vi "kSARegisterForData.vi"(0 "kSAComm ref in":refnum<k24>, 1 "Data Definitions":T1(array[cluster])) -> (2 "kSAComm ref out":refnum<k24>, 3 "Success":bool, 4 "Error":string)   [LabVIEW 2019]
doc: "Set up the kSA Data Store with the desired data items to retrieve when syncing data with the kSA Application."
uses:
  C:/Users/tim/Documents/kSAComm LabView Sample/kSACommInterface.dll
  kSACommInterface.dll
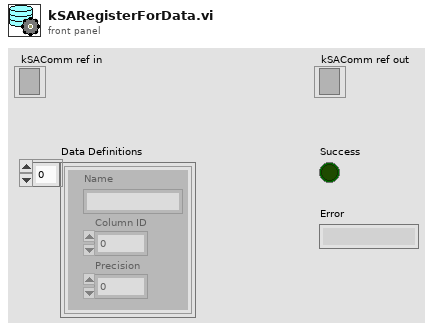
[diagram p1: front panel]
types:
  T1 = cluster{"Name":string, "Column ID":u32, "Precision":i32}[]
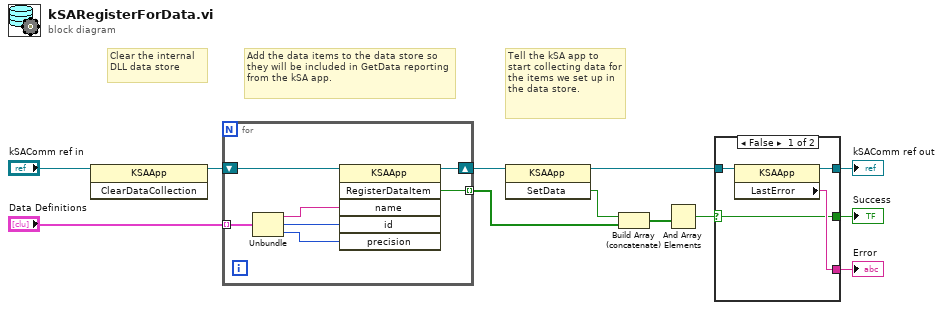
[diagram p0: block diagram]
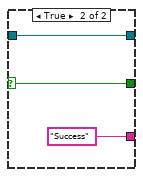
[diagram p2: hidden frame]
diagram:
  # "Add the data items to the data store so they will be included in GetData reporting from the kSA app."
  # "Clear the internal DLL data store"
  # "Tell the kSA app to start collecting data for the items we set up in the data store."
  n1 = invoke class="KSAApp" method="ClearDataCollection"(reference="kSAComm ref in") -> (reference out=w10:refnum<k24>)  [unwired: 2 in, 2 out]
  n2 = for {
    shift-right: [w14] -> w9
    shift-left: w10 -> [w15]
    tunnel: "Data Definitions" -> [w19] mode=indexing
    tunnel: [w13] -> w7 mode=indexing
    n3 = Unbundle(w19) -> ("Name"=w18:string, "Column ID"=w17:u32, "Precision"=w16:i32)
    n4 = invoke class="KSAApp" method="RegisterDataItem"(reference=w15, "name"=w18, "id"=w17, "precision"=w16) -> (reference out=w14:refnum<k24>, "RegisterDataItem"=w13:bool)  [unwired: 2 in, 4 out]
  }
  n5 = invoke class="KSAApp" method="SetData"(reference=w9) -> (reference out=w4:refnum<k24>, "SetData"=w8:bool)  [unwired: 2 in, 1 out]
  n6 = Build Array (concatenate)(w8, w7) -> (w6:bool[])
  n7 = And Array Elements(Boolean array=w6) -> (logical AND=w2:bool)
  n8 = case shown="False" w2 {
    selector: w2 -> [w20 w24]
    tunnel: [w23 "Success" ("LastError")] -> w5
    tunnel: w4 -> [w22 w25]
    tunnel: [w21 w25] -> w3
    tunnel: [w20 w24] -> w1
    frame False {
      n9 = property class="KSAApp"(reference=w22) -> (reference out=w21:refnum<k24>, "LastError"=w23:string)  [unwired: 1 in, 1 out]
    }
    frame True {
    }
  }
  "kSAComm ref out" <- w3
  "Success" <- w1
  "Error" <- w5
